vi "RSZVB Get Display Results State.vi"(8 "error in (no error)":errorcluster {"code" format="%.0x"}, 9 "Result Type (0: Phase Delay/El Length)":i32(ring) items=["Phase Delay/El Length", "Min/Max/Peak-Peak", "Mean/Std Dev", "RMS", "Gain/Slope/Flatness", "Compression Point"], 10 "Channel (Trace) (1)":i32=1, 11 "VISA session":refnum<visa-resource-name>) -> (0 "error out":errorcluster {"code" format="%.0x"}, 1 "Display Results":bool, 3 "dup VISA session":refnum<visa-resource-name>)   [LabVIEW 2011]
doc: "This VI returns the Phase Delay/El Length, Min/Max/Peak-Peak, Mean/Std Dev, RMS, Gain/Slope/Flatness or Compression Point results state.\n\nRemote-control command(s):\nCALCulate<Chn>:STATistics:EPDelay[:STATe]?\nCALCulate<Chn>:STATistics:MMPTpeak[:STATe]?\nCALCulate<Chn>:STATistics:MSTDdev[:STATe]?\nCALCulate<Chn>:STATistics:RMS[:STATe]?\nCALCulate<Chn>:STATistics:SFLatness[:STATe]?\nCALCulate<Chn>:STATistics:NLINear:COMP[:STATe]?"
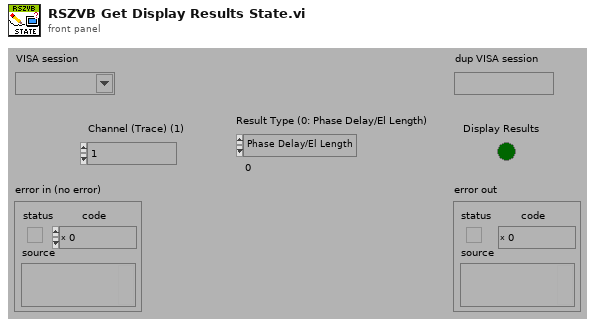
[diagram p1: front panel]
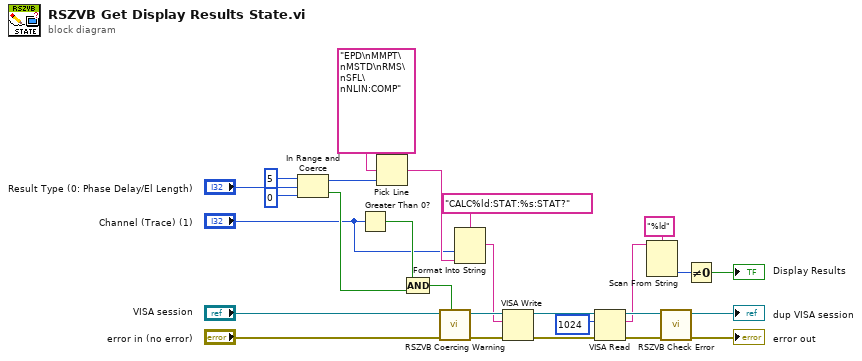
[diagram p0: block diagram]
diagram:
  n1 = In Range and Coerce(upper limit=5 ("lower limit"), x="Result Type (0: Phase Delay/El Length)", lower limit=0) -> (coerced(x)=w20:i32, In Range?=w18:bool)
  n2 = Greater Than 0?(x="Channel (Trace) (1)") -> (x > 0?=w19:bool)
  n3 = Pick Line(multi-line string="EPD\nMMPT\nMSTD\nRMS\nSFL\nNLIN:COMP", line index=w20) -> (output string=w23:string)  [unwired: 1 in]
  n4 = Compound Arithmetic op=AND(w19, w18) -> (w17:bool)
  n5 = call "RSZVB Coercing Warning.vi"("In Range?"=w17, "error in (no error)"="error in (no error)", "VISA session"="VISA session") -> ("error out"=w25:errorcluster, "dup VISA session"=w26:refnum<visa-resource-name>)  [unwired: 7 in]
  n6 = Format Into String(format string="CALC%ld:STAT:%s:STAT?", "Channel (Trace) (1)", w23) -> (resulting string=w24:string)  [unwired: 2 in, 1 out]
  n7 = VISA Write(VISA resource name=w26, write buffer=w24, error in (no error)=w25) -> (VISA resource name out=w6:refnum<visa-resource-name>, error out=w7:errorcluster)  [unwired: 1 out]
  n8 = VISA Read(VISA resource name=w6, byte count=u32 1024 ("byte count (0)"), error in (no error)=w7) -> (VISA resource name out=w11:refnum<visa-resource-name>, read buffer=w9:string, error out=w10:errorcluster)  [unwired: 1 out]
  n9 = Scan From String(format string="%ld", input string=w9) -> (output 1=w8:i32)  [unwired: 3 in, 3 out]
  n10 = call "RSZVB Check Error.vi"("error in (no error)"=w10, "VISA session"=w11) -> ("error out"=→"error out":errorcluster, "dup VISA session"=→"dup VISA session":refnum<visa-resource-name>)  [unwired: 8 in]
  n11 = Not Equal To 0?(x=w8) -> (x != 0?=→"Display Results":bool)
